vi "CalcPercentFromUndesired.vi"(6 "Target \nOutput":i32, 8 "Delay Time (s)":dbl=0.05, 9 "Error In":errorcluster, 10 "Arduino Digital Outputs":u8[](array[numeric]), 11 "LINX Resource In":T1) -> (1 "Positive values":bool, 2 "[unwanted/total]^2":dbl)   [LabVIEW 2018]
uses:
  <vilib>/MakerHub/LINX/Private/Type Defs/LINX Ref.ctl
  <vilib>/MakerHub/LINX/Private/Type Defs/Platform.ctl
  <vilib>/MakerHub/LINX/Private/Type Defs/Interface.ctl
  <vilib>/MakerHub/LINX/Private/Device/Type Defs/LINX Device Config.ctl
  <vilib>/MakerHub/LINX/Private/Device/Type Defs/TCP Config.ctl
  <vilib>/MakerHub/LINX/Private/Device/Type Defs/Channels.ctl
  <vilib>/MakerHub/LINX/Public/Peripherals/Digital/Digital Write N Chans.vi
  <vilib>/MakerHub/LINX/Private/Local IO/LinxDigitalWrite.vi
  <vilib>/MakerHub/LINX/Public/Utilities/Check Channel.vi
  GlobalVariables/GlobalStop.vi
  GlobalVariables/WaveformCharGlobal.vi
  <vilib>/MakerHub/LINX/Private/Utilties/Generate Error.vi
  <vilib>/express/express arith-compare/Formula/XNode/ExpressFormulaBlockNode.xnode
  <vilib>/MakerHub/LINX/LMH-LINX.lvlib
  <vilib>/MakerHub/LINX/Private/Device/Device.lvlib
panel:
  out "Error Out":errorcluster
  out "LINX Resource":T1
  out "Current output (mA)":dbl
  in  "Fixed Resistor":dbl=350.0
  out "MUX channel":i32
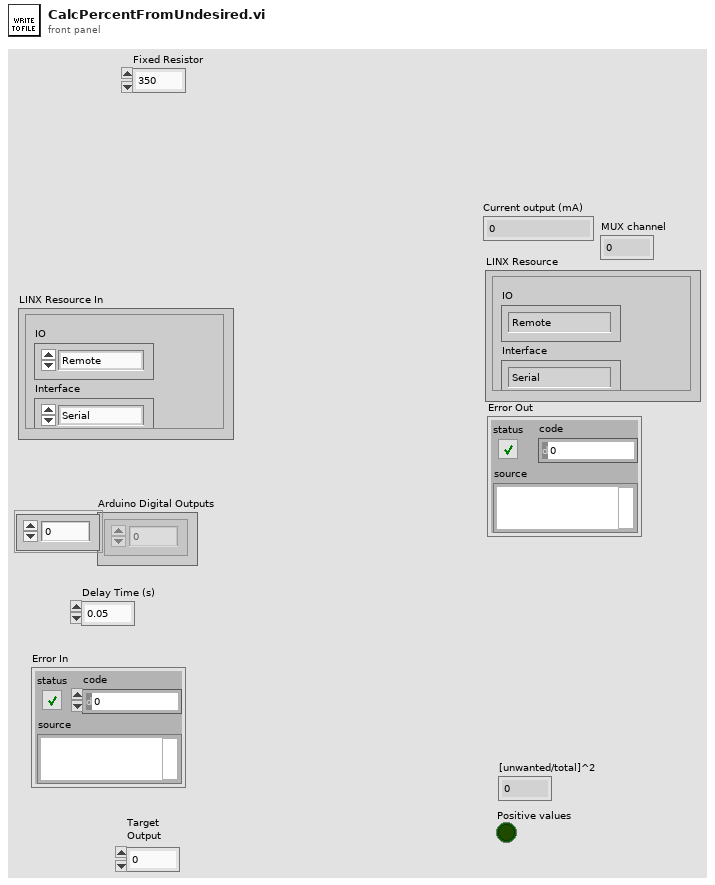
[diagram p1: front panel]
types:
  T1 = typedef "LMH-LINX.lvlib/LINX Ref.ctl" = cluster{"IO":T2, "Interface":T3, "LINX Device Config":T4}
  T2 = typedef "LMH-LINX.lvlib/Platform.ctl" = enum16{"Remote", "Local"}
  T3 = typedef "LMH-LINX.lvlib/Interface.ctl" = enum16{"Serial", "TCP"}
  T4 = typedef "LMH-LINX.lvlib/Device.lvlib/LINX Device Config.ctl" = cluster{"Interface":T3, "COM Port":refnum<visa-resource-name>, "TCP Configuration":T5, "Device Family":u8, "Device ID":u8, "Device Name":string, "TCP Ref":refnum<k5>, "Channels":T6}
  T5 = typedef "LMH-LINX.lvlib/Device.lvlib/TCP Config.ctl" = cluster{"IP Address":string, "Port":u16}
  T6 = typedef "LMH-LINX.lvlib/Channels.ctl" = cluster{"DI":u8[], "DO":u8[], "AI":u8[], "AO":u8[], "PWM":u8[], "QE":u8[], "UART":u8[], "I2C 2":u8[], "SPI":u8[], "CAN":u8[], "Servo":u8[], "AI Ref (V)":dbl, "AI Resolution (Bits)":u8, "AO Ref (V)":dbl, "AO Resolution (Bits)":u8}
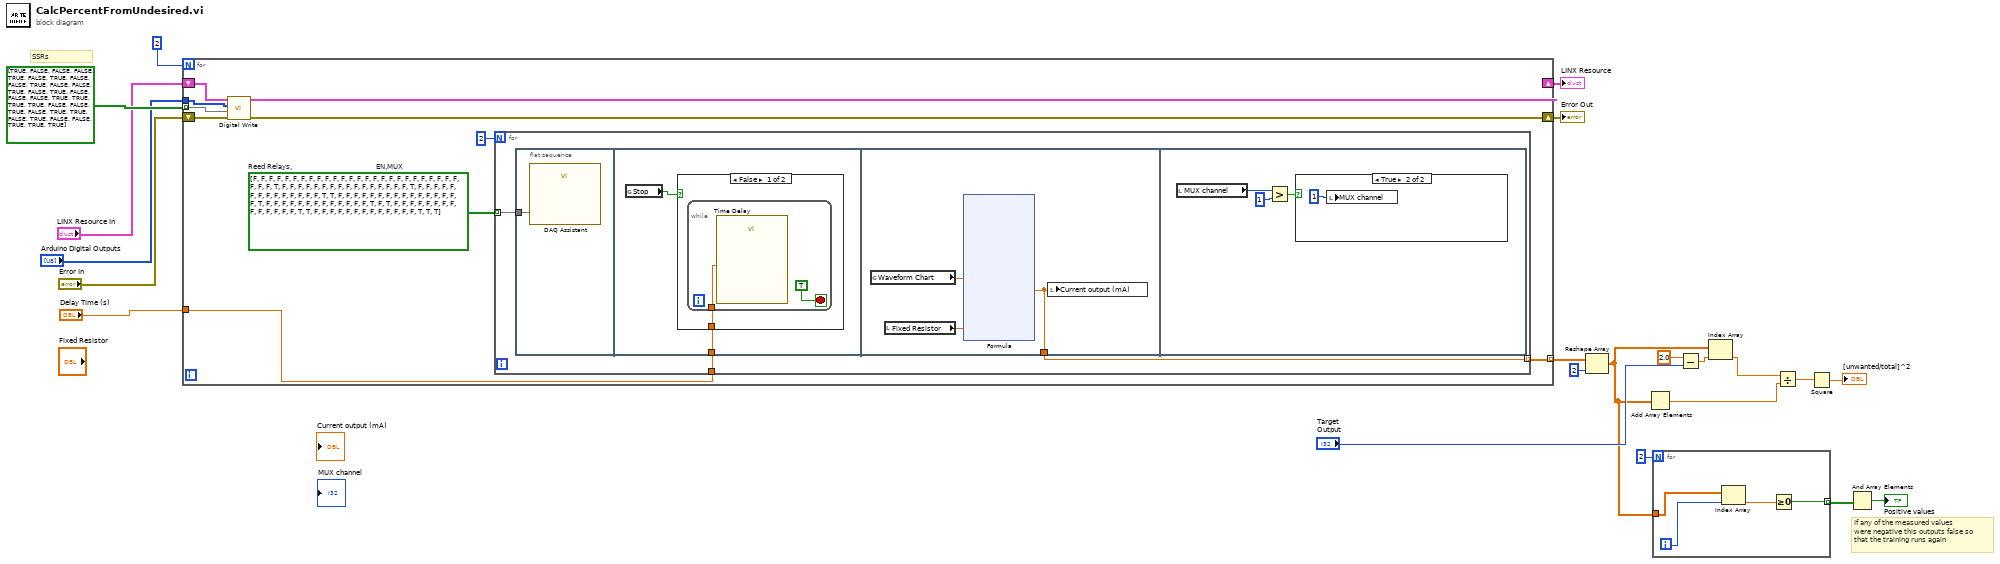
[diagram p0: block diagram]
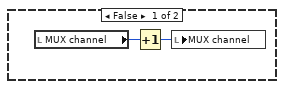
[diagram p3: hidden frame]
diagram:
  # "If any of the measured values\nwere negative this outputs false so \nthat the training runs again"
  # "SSRs"
  n1 = for {
    N: 2 -> [_]
    shift-right: [w28] -> w18
    shift-left: "Error In" -> [w30]
    shift-right: [w27] -> w19
    shift-left: "LINX Resource In" -> [w29]
    tunnel: [w26] -> w13 mode=indexing
    tunnel: bool[][] [[TRUE, FALSE, FALSE, FALSE, TRUE], [FALSE, TRUE, FALSE, FALSE, TRUE], [FALSE, FALSE, TRUE, FALSE, TRUE], [FALSE, FALSE, FALSE, TRUE, TRUE], [TRUE, TRUE, FALSE, FALSE, TRUE], [FALSE, TRUE, TRUE, FALSE, TRUE], [FALSE, FALSE, TRUE, TRUE, TRUE]] ("Values") -> [w25] mode=indexing
    tunnel: "Delay Time (s)" -> [w23]
    tunnel: "Arduino Digital Outputs" -> [w22]
    w31 = bool[][] [[FALSE, FALSE, FALSE, FALSE, FALSE, FALSE, FALSE, FALSE, FALSE, FALSE, FALSE, FALSE, FALSE, FALSE, FALSE, FALSE], [FALSE, FALSE, FALSE, FALSE, FALSE, FALSE, FALSE, FALSE, FALSE, FALSE, FALSE, FALSE, FALSE, TRUE, FALSE, FALSE], [FALSE, FALSE, FALSE, FALSE, FALSE, FALSE, FALSE, FALSE, FALSE, FALSE, FALSE, FALSE, FALSE, FALSE, TRUE, FALSE], [FALSE, FALSE, FALSE, FALSE, FALSE, FALSE, FALSE, FALSE, FALSE, FALSE, FALSE, FALSE, FALSE, TRUE, TRUE, FALSE], [FALSE, FALSE, FALSE, FALSE, FALSE, FALSE, FALSE, FALSE, FALSE, FALSE, FALSE, FALSE, FALSE, FALSE, FALSE, TRUE], [FALSE, FALSE, FALSE, FALSE, FALSE, FALSE, FALSE, FALSE, FALSE, FALSE, FALSE, FALSE, FALSE, TRUE, FALSE, TRUE], [FALSE, FALSE, FALSE, FALSE, FALSE, FALSE, FALSE, FALSE, FALSE, FALSE, FALSE, FALSE, FALSE, FALSE, TRUE, TRUE], [FALSE, FALSE, FALSE, FALSE, FALSE, FALSE, FALSE, FALSE, FALSE, FALSE, FALSE, FALSE, FALSE, TRUE, TRUE, TRUE]]  # Reed Relays,                                          EN,MUX
    n2 = call-poly <vilib>:"Digital Write.vi"("Error In"=w30, "Values"=w25, "DO Channels"=w22, "LINX Resource"=w29) -> ("Error Out"=w28:errorcluster, "LINX Resource"=w27:T1)  [unwired: 6 in]
    n3 = for {
      N: 2 -> [_]
      tunnel: w31 -> [w34] mode=indexing
      tunnel: [w33] -> w26 mode=indexing
      tunnel: w23 -> [w32]
      n4 = flat-sequence {
        tunnel: w34 -> [w35]
        tunnel: w32 -> [w36]
        tunnel: [w42] -> w33
        frame #0 {
          n5 = call "DAQ Assistant"("data"=w35) -> ()  [unwired: 17 in, 2 out]
        }
        frame #1 {
          n6 = global read "GlobalStop.vi" "Stop"() -> (w37:bool)
          n7 = case shown="False" w37 {
            tunnel: w36 -> [w38 _]
            frame False {
              n8 = while {
                tunnel: w38 -> [w39]
                stop <- TRUE stop-if-true
                n9 = call "Time Delay"("Delay Time (s)"=w39) -> ()  [unwired: 10 in, 1 out]
              }
            }
            frame True {
            }
          }
        }
        frame #2 {
          n10 = global read "WaveformCharGlobal.vi" "Waveform Chart"() -> (w41:dbl)
          n11 = local read "Fixed Resistor"() -> (w43:dbl)
          n12 = xnode "Formula"("X1"=w41, "X2"=w43) -> ("Result"=w42:dbl)  [unwired: 1 in, 1 out]
          n13 = local write "Current output (mA)"(w42) -> ()
        }
        frame #3 {
          n14 = local read "MUX channel"() -> (w55:i32)
          n15 = Greater?(x=w55, y=1) -> (0:w56:bool)
          n16 = case shown="True" w56 {
            frame False {
              n17 = local read "MUX channel"() -> (w58:i32)
              n18 = Increment(x=w58) -> (x+1=w57:i32)
              n19 = local write "MUX channel"(w57) -> ()
            }
            frame True {
              n20 = local write "MUX channel"(1 ("MUX channel")) -> ()
            }
          }
        }
      }
    }
  }
  "LINX Resource" <- w19
  "Error Out" <- w18
  n21 = Reshape Array(w13, 2 ("dimension size")) -> (w3:dbl[])
  n22 = Add Array Elements(numeric array=w3) -> (sum=w7:dbl)
  n23 = for {
    N: 2 -> [_]
    tunnel: w3 -> [w63]
    tunnel: [w60] -> w1 mode=indexing
    i -> [w62]
    n24 = Index Array(array=w63, index=w62) -> (element=w61:dbl)
    n25 = Greater Or Equal To 0?(x=w61) -> (x >= 0?=w60:bool)
  }
  n26 = Subtract(x=2.0, y="Target \nOutput") -> (x-y=w11:dbl)
  n27 = Index Array(array=w3, index=w11) -> (element=w8:dbl)
  n28 = Divide(x=w8, y=w7) -> (x/y=w6:dbl)
  n29 = Square(x=w6) -> (x^2=→"[unwanted/total]^2":dbl)
  n30 = And Array Elements(Boolean array=w1) -> (logical AND=→"Positive values":bool)
